vi "Set Level.vi"(7 "Output Channel":T1, 8 "error in (no error)":errorcluster, 10 "Level (V)":dbl, 11 "VISA Refnum in":refnum<visa-resource-name>) -> (0 "error out":errorcluster, 3 "VISA Refnum out":refnum<visa-resource-name>)   [LabVIEW 2016, in "RP100.lvclass"]
uses:
  RP100.lvclass
  Typedefs/Output Channel--Enum.ctl
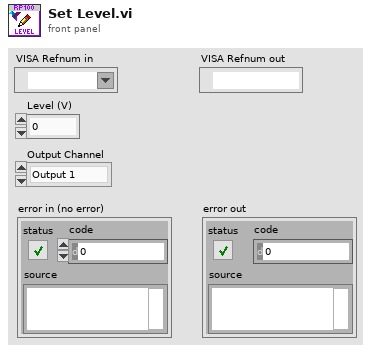
[diagram p1: front panel]
types:
  T1 = typedef "RP100.lvclass/Output Channel--Enum.ctl" = enum16{"Output 1", "Output 2"}
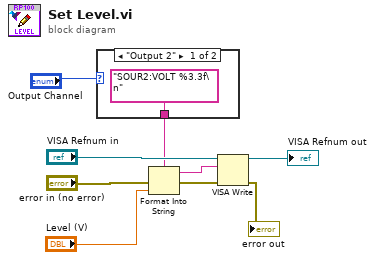
[diagram p0: block diagram]
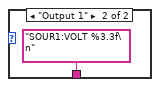
[diagram p2: hidden frame]
diagram:
  n1 = case shown="\"Output 2\"" "Output Channel" {
    tunnel: ["SOUR2:VOLT %3.3f\n" ("format string") "SOUR1:VOLT %3.3f\n" ("format string")] -> w1
    frame "Output 2" {
    }
    frame "Output 1" {
    }
  }
  n2 = Format Into String(format string=w1, error in="error in (no error)", "Level (V)") -> (resulting string=w6:string, error out=w3:errorcluster)  [unwired: 1 in]
  n3 = VISA Write(VISA resource name="VISA Refnum in", write buffer=w6, error in (no error)=w3) -> (VISA resource name out=→"VISA Refnum out":refnum<visa-resource-name>, error out=→"error out":errorcluster)  [unwired: 1 out]
